vi "Create.vi"(8 "error in (no error)":errorcluster, 11 "Port":string) -> (0 "error out":errorcluster, 3 "VisaResource out":refnum<class "VisaResource.lvclass">)   [LabVIEW 2020, in "VisaResource.lvclass"]
uses:
  VisaResource.lvclass
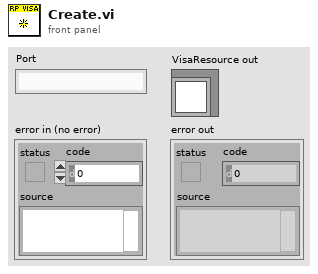
[diagram p1: front panel]
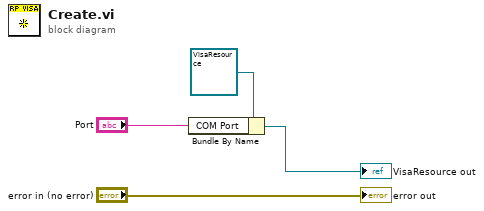
[diagram p0: block diagram]
diagram:
  n1 = Bundle By Name(cluster=refnum<class "VisaResource.lvclass"> refnum ("VisaResource out"), "COM Port"="Port") -> (→"VisaResource out":refnum<class "VisaResource.lvclass">)
  "error out" <- "error in (no error)"
